vi "CheckHoldLotSheet.vi"() -> ()   [LabVIEW 2012]
uses:
  <vilib>/Utility/NIReport.llb/NI_report.lvclass
  <vilib>/addons/_office/excel.llb/Excel Get Data (str).vi
  <vilib>/Utility/NIReport.llb/Excel/NI_Excel.lvclass
  <vilib>/addons/_office/NI_ReportGenerationToolkit.lvlib
  <vilib>/Utility/SMTP/NI_SMTPEmail.lvlib
panel:
  out "Numeric":i32
  out "data":string
  out "step":string
  out "spreadsheet string":string
  out "output array":string[](array[string])
  out "array":string[](array[string])
  out "error out":errorcluster
  in  "start (0, 0)":cluster{"start row":i32, "start column":i32}
  out "row":i32
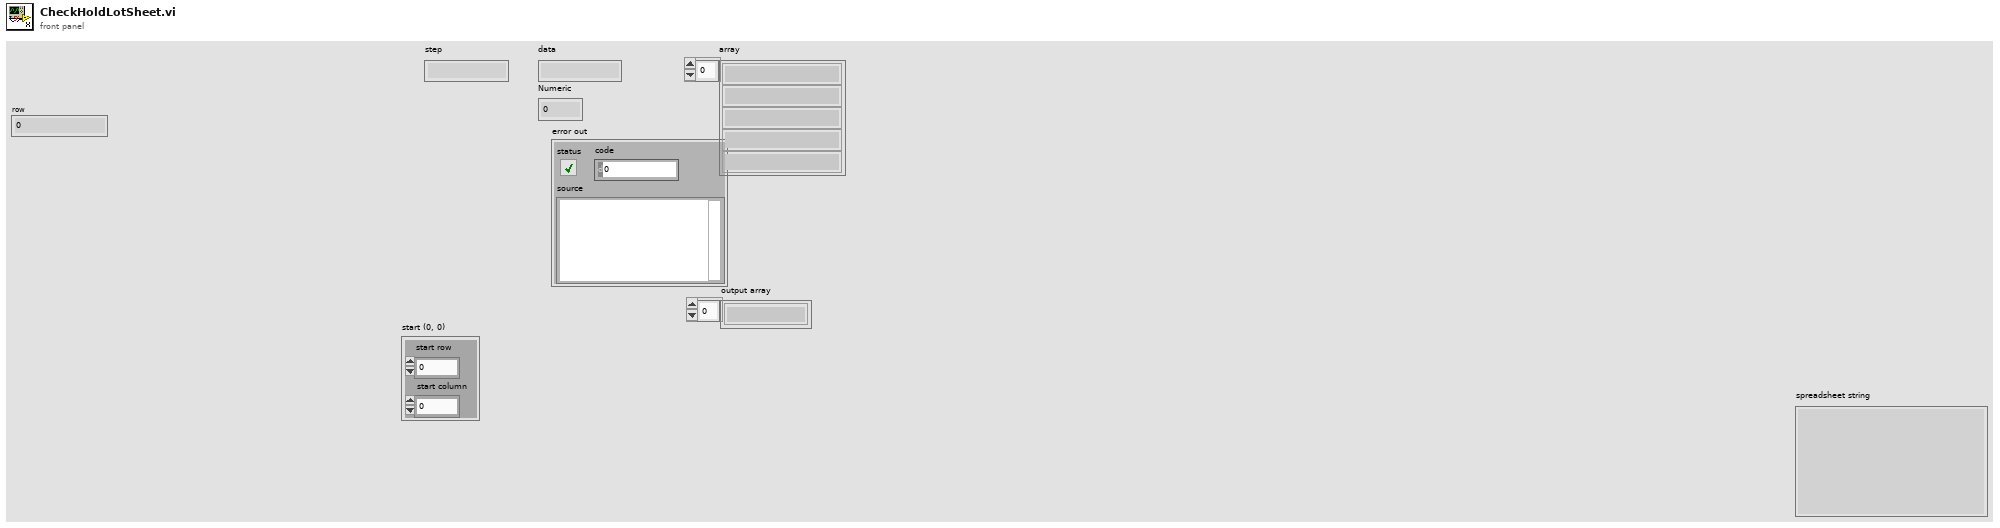
[diagram p1: front panel]
types:
  T1 = enum16{"Standard Report", "HTML", "Word", "Excel"}
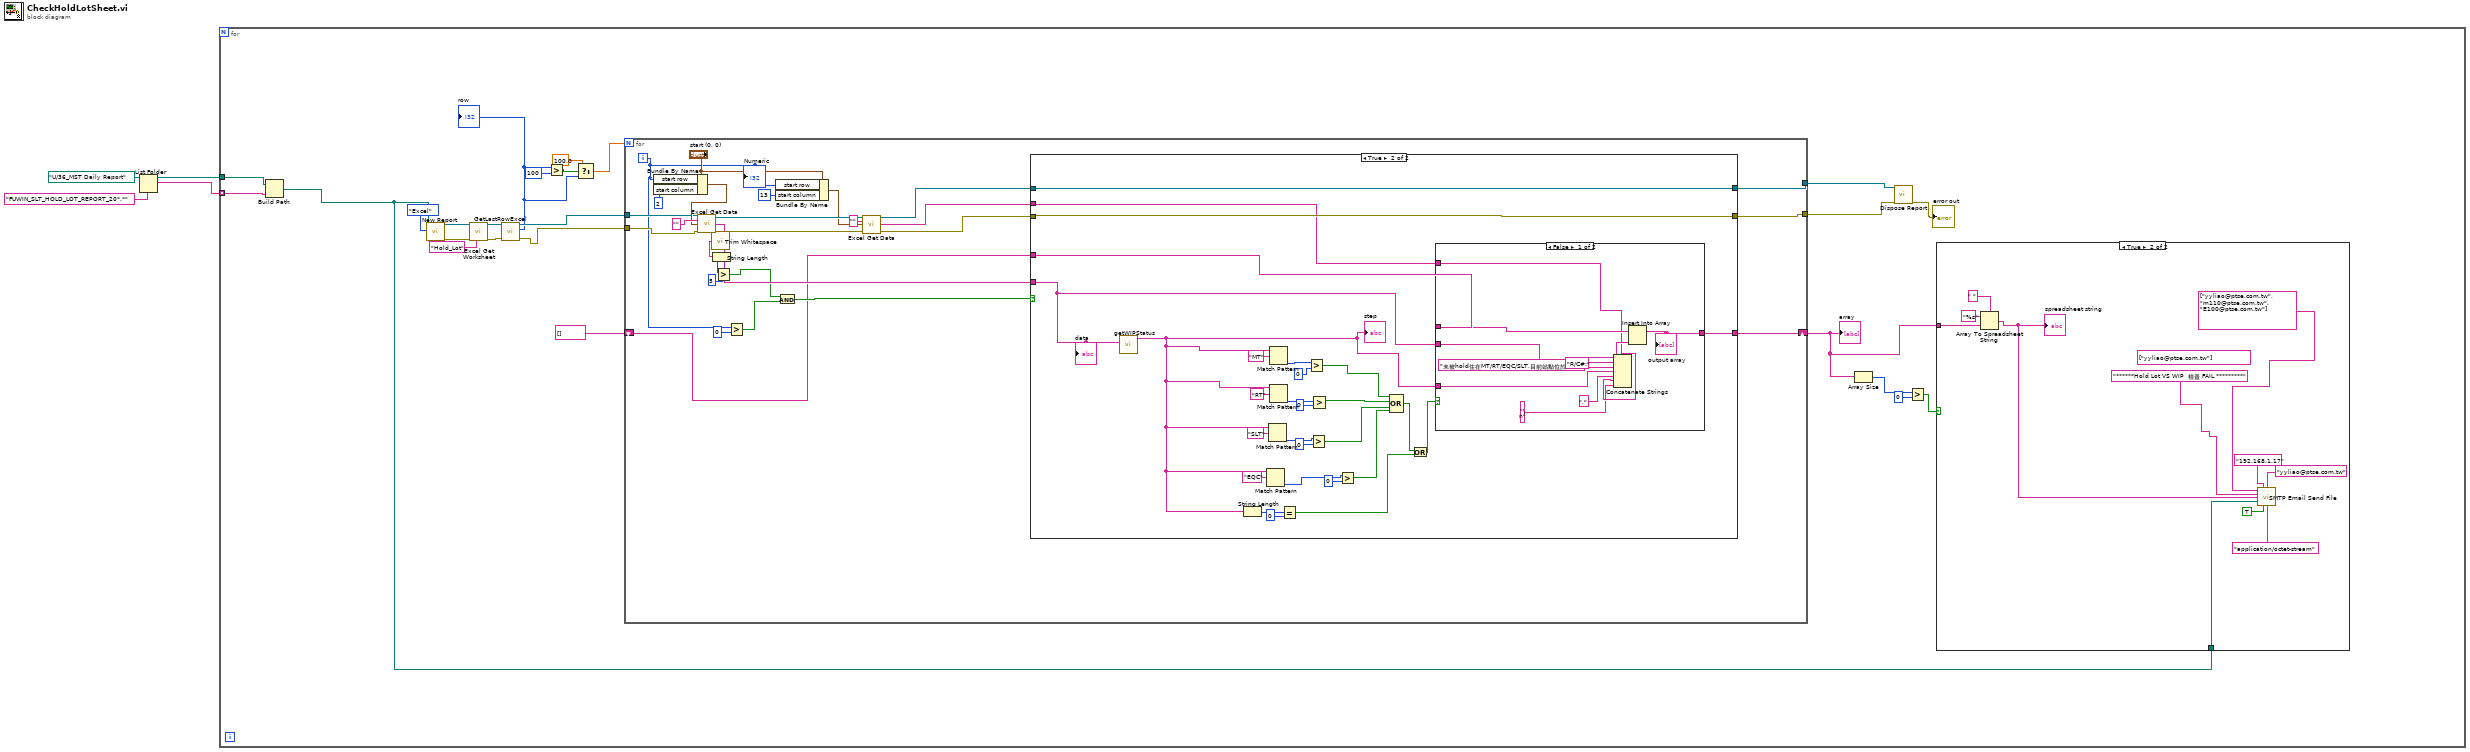
[diagram p0: block diagram]
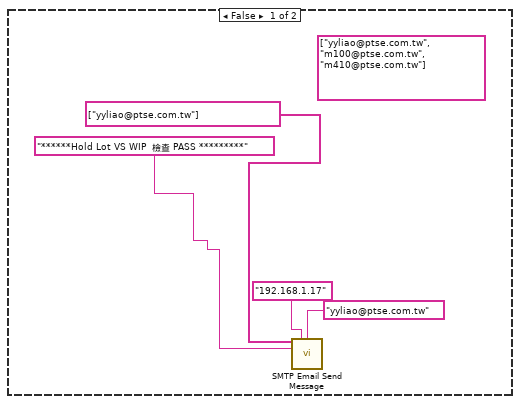
[diagram p2: hidden frame]
diagram:
  n1 = List Folder(path=path "U:/36_MST Daily Report", pattern="FUWIN_SLT_HOLD_LOT_REPORT_20*.*") -> (path out=w2:path, filenames=w1:string[])  [unwired: 2 in, 2 out]
  n2 = for {
    tunnel: w2 -> [w10]
    tunnel: w1 -> [w9] mode=indexing
    n3 = Build Path(base path=w10, name or relative path=w9) -> (appended path=w8:path)
    n4 = call <vilib>:"New Report.vi"("report type"=T1."Excel" ("Report Type"), "template (empty)"=w8) -> ("report out"=w27:refnum<class "NI_report.lvclass">, "error out"=w26:errorcluster)  [unwired: 12 in]
    n5 = call <vilib>:"Excel Get Worksheet.vi"("report in"=w27, "error in (no error)"=w26, "name (\"\")"="Hold_Lot" ("name (\"\")")) -> ("report out"=w25:refnum<class "NI_report.lvclass">, "error out"=w24:errorcluster)  [unwired: 11 in]
    n6 = call "GetLastRowExcel.vi"("error in (no error)"=w24, "report in"=w25) -> ("error out"=w23:errorcluster, "row"=w16:i32, "report out"=w22:refnum<class "NI_report.lvclass">)  [unwired: 7 in]
    "row" <- w16
    n7 = Greater?(x=w16, y=100) -> (0:w18:bool)
    n8 = Select(t=100.0, s=w18, f=w16) -> (s? t:f=w15:dbl)
    n9 = for {
      N: w15 -> [_]
      tunnel: w22 -> [w62]
      tunnel: w23 -> [w61]
      tunnel: [w54] -> w7
      tunnel: [w65] -> w6
      shift-right: [w56] -> w11
      shift-left: string[] [] ("array") -> [w55]
      i -> [w48]
      n10 = Bundle By Name(cluster="start (0, 0)", "start row"=w48, "start column"=2) -> (w64:cluster{"start row":i32, "start column":i32})
      n11 = call-poly <vilib>:"Excel Get Data.vi"("report in"=w62, "data type"="", "start (0, 0)"=w64, "error in (no error)"=w61) -> ("report out"=w51:refnum<class "NI_report.lvclass">, "data"=w63:string, "error out"=w53:errorcluster)  [unwired: 9 in]
      n12 = call <vilib>:"Trim Whitespace.vi"("string"=w63) -> ("trimmed string"=w67:string)  [unwired: 1 in]
      n13 = String Length(string=w67) -> (length=w66:i32)
      n14 = Greater?(x=w66, y=5) -> (0:w58:bool)
      n15 = Greater?(x=w48, y=0) -> (0:w59:bool)
      n16 = Bundle By Name(cluster="start (0, 0)", "start row"=w48, "start column"=13) -> (w50:cluster{"start row":i32, "start column":i32})
      n17 = And(x=w58, y=w59) -> (x .and. y?=w57:bool)
      n18 = call-poly <vilib>:"Excel Get Data.vi"("report in"=w51, "data type"="", "start (0, 0)"=w50, "error in (no error)"=w53) -> ("report out"=w44:refnum<class "NI_report.lvclass">, "data"=w45:string, "error out"=w52:errorcluster)  [unwired: 9 in]
      n19 = case shown="True" w57 {
        tunnel: w63 -> [_ w88]
        tunnel: w44 -> [w71 w81]
        tunnel: w52 -> [w73 w101]
        tunnel: [w71 w81] -> w54
        tunnel: [w73 w101] -> w65
        tunnel: [w72 w87] -> w56
        tunnel: w55 -> [w72 w86]
        tunnel: w45 -> [_ w80]
        frame False {
        }
        frame True {
          n20 = call "getWIPStatus.vi"("Lotno"=w88) -> ("step"=w79:string)  [unwired: 9 in, 1 out]
          "step" <- w79
          n21 = String Length(string=w79) -> (length=w78:i32)
          n22 = Match Pattern(string=w79, regular expression="EQC") -> (offset past match=w83:i32)  [unwired: 1 in, 3 out]
          n23 = Match Pattern(string=w79, regular expression="SLT") -> (offset past match=w93:i32)  [unwired: 1 in, 3 out]
          n24 = Match Pattern(string=w79, regular expression="MT") -> (offset past match=w97:i32)  [unwired: 1 in, 3 out]
          n25 = Match Pattern(string=w79, regular expression="RT") -> (offset past match=w95:i32)  [unwired: 1 in, 3 out]
          n26 = Equal?(x=w78, y=0) -> (x = y?=w75:bool)
          n27 = Greater?(x=w97, y=0) -> (0:w91:bool)
          n28 = Greater?(x=w93, y=0) -> (0:w89:bool)
          n29 = Greater?(x=w95, y=0) -> (0:w90:bool)
          n30 = Greater?(x=w83, y=0) -> (0:w82:bool)
          n31 = Compound Arithmetic op=OR(w91, w90, w89, w82) -> (w76:bool)
          n32 = Or(x=w76, y=w75) -> (x .or. y?=w74:bool)
          n33 = case shown="False" w74 {
            tunnel: w88 -> [w108 _]
            tunnel: [w111 w112] -> w87
            tunnel: w86 -> [w110 w112]
            tunnel: w79 -> [w105 _]
            tunnel: w80 -> [w103 _]
            frame False {
              n34 = Concatenate Strings("R/C#:" ("string"), w108, "未被hold住在MT/RT/EQC/SLT,目前站點位於" ("string"), w105, "," ("string"), w103, "\n" ("string")) -> (w106:string)
              n35 = Insert Into Array(array=w110, new element=w106) -> (w111:string[])  [unwired: 1 in]
              "output array" <- w111
            }
            frame True {
            }
          }
          "data" <- w88
        }
      }
      "Numeric" <- w48
    }
    "array" <- w11
    n36 = Array Size(array=w11) -> (size(s)=w14:i32)
    n37 = call-dynamic "Dispose Report.vi"("report in"=w7, "error in (no error)"=w6) -> ("error out"=→"error out":errorcluster)  [unwired: 13 in]
    n38 = Greater?(x=w14, y=0) -> (0:w12:bool)
    n39 = case shown="True" w12 {
      tunnel: w11 -> [_ w37]
      tunnel: w8 -> [_ w34]
      frame False {
        (unwired) string[] ["yyliao@ptse.com.tw", "m100@ptse.com.tw", "m410@ptse.com.tw"] ("recipients")
        n40 = call <vilib>:"SMTP Email Send Message.vi"("recipients"=string[] ["yyliao@ptse.com.tw"], "mail server"="192.168.1.17", "return address"="yyliao@ptse.com.tw", "subject ([No Subject])"="******Hold Lot VS WIP  檢查 PASS *********") -> ()  [unwired: 10 in, 2 out]
      }
      frame True {
        (unwired) string[] ["yyliao@ptse.com.tw"] ("recipients")
        n41 = Array To Spreadsheet String(delimiter (Tab)=" ", array=w37, 3:"%s" ("format string")) -> (spreadsheet string=w36:string)
        "spreadsheet string" <- w36
        n42 = call <vilib>:"SMTP Email Send File.vi"("recipients"=string[] ["yyliao@ptse.com.tw", "m110@ptse.com.tw", "E100@ptse.com.tw"], "mail server"="192.168.1.17", "return address"="yyliao@ptse.com.tw", "subject ([No Subject])"="******Hold Lot VS WIP  檢查 FAIL *********", "message"=w36, "file path"=w34, "binary? (F)"=TRUE, "MIME content-type (application/octet-stream)"="application/octet-stream") -> ()  [unwired: 6 in, 2 out]
      }
    }
  }
